vi "MSEncoder Case-44-UpdDO.vi"(8 "error in (no error)":errorcluster, 9 "ParamValIn":variant, 11 "MSEncoder in":refnum<class "MSEncoder.lvclass">) -> (0 "error out":errorcluster, 3 "MSEncoder out":refnum<class "MSEncoder.lvclass">)   [LabVIEW 2018, in "MSEncoder.lvclass"]
uses:
  MSEncoder.lvclass
  Ctl/MSEditorParam updDO.ctl
  MSEncoder.lvclass/MSEncoder.ctl
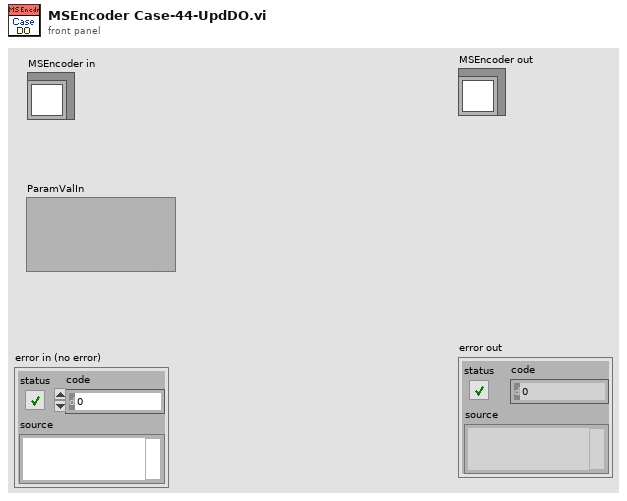
[diagram p1: front panel]
types:
  T1 = typedef "MSEditorParam updDO.ctl" = cluster{"func":u32[], "val":bool[]}
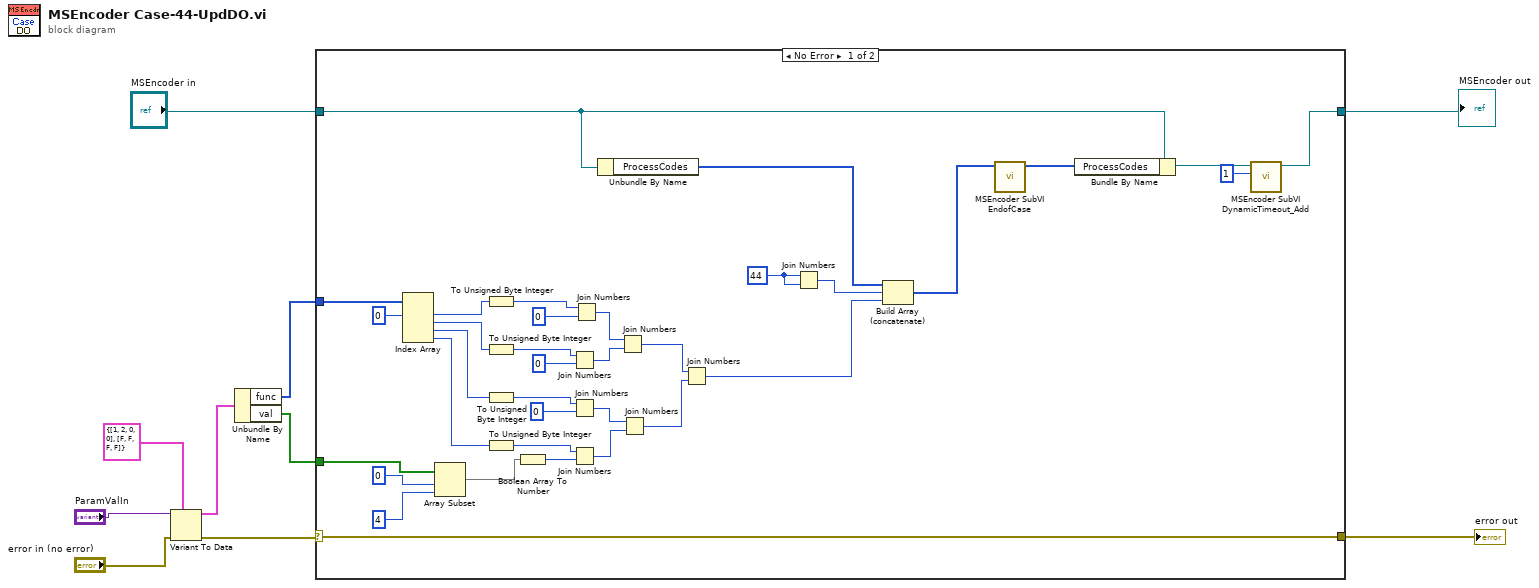
[diagram p0: block diagram]
diagram:
  n1 = Variant To Data(error in="error in (no error)", type=T1 {"func"=[1, 2, 0, 0], "val"=[FALSE, FALSE, FALSE, FALSE]} ("ParamValueOutput"), Variant="ParamValIn") -> (data=w3:T1, error out=w2:errorcluster)
  n2 = Unbundle By Name(w3) -> ("func"=w9:u32[], "val"=w8:bool[])
  n3 = case shown="No Error" w2 {
    selector: w2 -> [w44 w47]
    tunnel: "MSEncoder in" -> [w43 w46]
    tunnel: [w44 w47] -> w10
    tunnel: [w12 w46] -> w7
    tunnel: w9 -> [w14 _]
    tunnel: w8 -> [w15 _]
    frame No Error {
      w41 = u32 44
      n4 = Index Array(array=w14, index #1=0 ("index")) -> (element #1=w23:u32, element #2=w21:u32, element #3=w20:u32, element #4=w19:u32)  [unwired: 3 in]
      n5 = Array Subset(array=w15, index=0, length=4) -> (w18:bool[])
      n6 = To Unsigned Byte Integer(number=w23) -> (unsigned 8bit integer=w38:u8)
      n7 = To Unsigned Byte Integer(number=w21) -> (unsigned 8bit integer=w35:u8)
      n8 = To Unsigned Byte Integer(number=w20) -> (unsigned 8bit integer=w33:u8)
      n9 = To Unsigned Byte Integer(number=w19) -> (unsigned 8bit integer=w32:u8)
      n10 = Boolean Array To Number(Boolean array=w18) -> (number=w31:u8)
      n11 = Join Numbers(hi=w35, lo=u8 0) -> ((hi.lo)=w27:u16)
      n12 = Join Numbers(hi=w33, lo=u8 0) -> ((hi.lo)=w29:u16)
      n13 = Join Numbers(hi=w32, lo=w31) -> ((hi.lo)=w30:u16)
      n14 = Join Numbers(hi=w38, lo=u8 0) -> ((hi.lo)=w28:u16)
      n15 = Unbundle By Name(w43) -> ("ProcessCodes"=w45:u64[])
      n16 = Join Numbers(hi=w28, lo=w27) -> ((hi.lo)=w26:u32)
      n17 = Join Numbers(hi=w29, lo=w30) -> ((hi.lo)=w25:u32)
      n18 = Join Numbers(hi=w26, lo=w25) -> ((hi.lo)=w24:u64)
      n19 = Join Numbers(hi=w41, lo=w41) -> ((hi.lo)=w40:u64)
      n20 = Build Array (concatenate)(w45, w40, w24) -> (w39:u64[])
      n21 = call "MSEncoder SubVI EndofCase.vi"("Case codes"=w39) -> ("Case codes with end"=w42:u64[])  [unwired: 9 in, 1 out]
      n22 = Bundle By Name(cluster=w43, "ProcessCodes"=w42) -> (w13:refnum<class "MSEncoder.lvclass">)
      n23 = call "MSEncoder SubVI DynamicTimeout_Add.vi"("Timeout_ms"=1, "MSEncoder"=w13) -> ("MSEncoder"=w12:refnum<class "MSEncoder.lvclass">)  [unwired: 8 in, 1 out]
    }
    frame Error {
    }
  }
  "error out" <- w10
  "MSEncoder out" <- w7
